vi "RSToutputWithUpDown.vi"(6 "RST Motor Constants":T1={"Pitch Gain (2*pi/enc)"=1.0, "Output Sign"=[1.0, -1.0, 1.0], "Phase Offset (rad)"=0.0, "Saturation"=32000.0}, 8 "flip Z":bool, 9 "Encoder Position":dbl, 10 "Z Command":dbl, 11 "X Command":dbl) -> (1 "Coerced?":bool, 3 "Control":dbl[](array[numeric]))   [LabVIEW 2011, in "kevLib2011.lvlib"]
uses:
  kevLib2011.lvlib
  RSTtypeDef.ctl
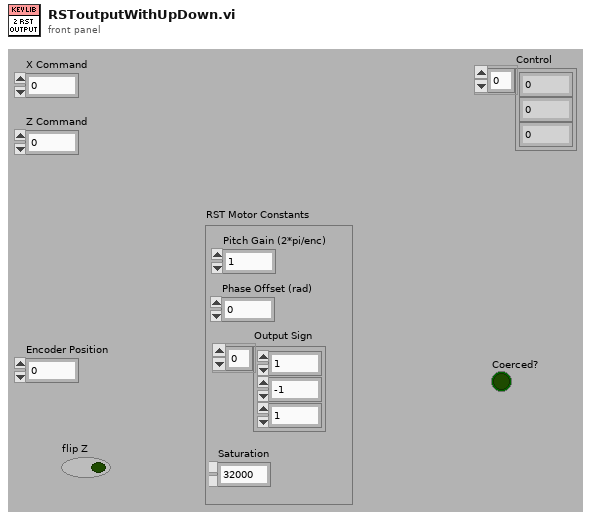
[diagram p1: front panel]
types:
  T1 = typedef "kevLib2011.lvlib/RSTtypeDef.ctl" = cluster{"Pitch Gain (2*pi/enc)":dbl, "Output Sign":dbl[], "Phase Offset (rad)":dbl, "Saturation":dbl}
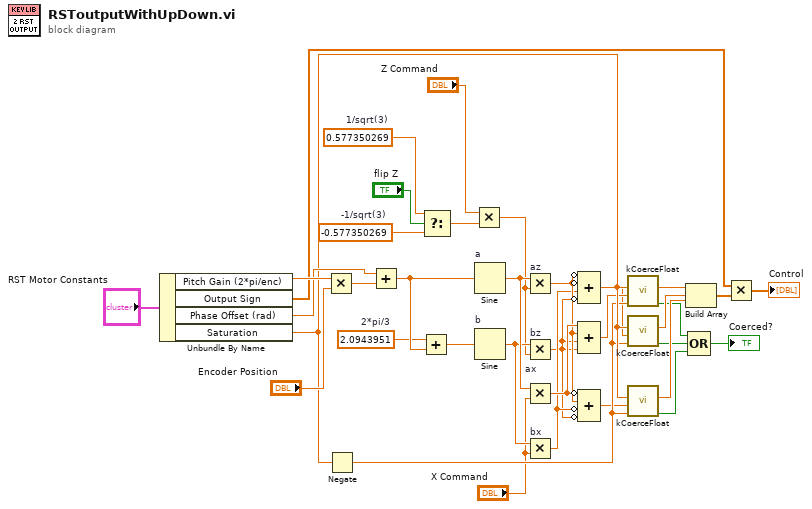
[diagram p0: block diagram]
diagram:
  w5 = -0.577350269  # -1/sqrt(3)
  w6 = 0.577350269  # 1/sqrt(3)
  w20 = 2.0943951  # 2*pi/3
  n1 = Unbundle By Name("RST Motor Constants") -> ("Pitch Gain (2*pi/enc)"=w34:dbl, "Output Sign"=w17:dbl[], "Phase Offset (rad)"=w32:dbl, "Saturation"=w24:dbl)
  n2 = Multiply(x=w34, y="Encoder Position") -> (x*y=w33:dbl)
  n3 = Negate(x=w24) -> (-x=w23:dbl)
  n4 = Add(x=w32, y=w33) -> (x+y=w22:dbl)
  n5 = Add(x=w20, y=w22) -> (x+y=w21:dbl)
  n6 = Select(t=w6, s="flip Z", f=w5) -> (s? t:f=w4:dbl)
  n7 = Multiply(x="Z Command", y=w4) -> (x*y=w12:dbl)
  n8 = Sine "a"(x=w22) -> (sin(x)=w15:dbl)
  n9 = Sine "b"(x=w21) -> (sin(x)=w14:dbl)
  n10 = Multiply "az"(x=w15, y=w12) -> (x*y=w10:dbl)
  n11 = Multiply "bz"(x=w14, y=w12) -> (x*y=w8:dbl)
  n12 = Multiply "ax"(x=w15, y="X Command") -> (x*y=w11:dbl)
  n13 = Multiply "bx"(x=w14, y="X Command") -> (x*y=w9:dbl)
  n14 = Compound Arithmetic op=ADD(invert w10, invert w10, w9, invert w8) -> (w2:dbl)
  n15 = Compound Arithmetic op=ADD(w11, w10, w8, w8) -> (w3:dbl)
  n16 = Compound Arithmetic op=ADD(invert w11, w10, invert w9, invert w8) -> (w1:dbl)
  n17 = call "kCoerceFloat.vi"("lower"=w23, "input"=w3, "upper"=w24) -> ("coerced?"=w28:bool, "output"=w31:dbl)  [unwired: 7 in]
  n18 = call "kCoerceFloat.vi"("lower"=w23, "input"=w2, "upper"=w24) -> ("coerced?"=w27:bool, "output"=w30:dbl)  [unwired: 7 in]
  n19 = call "kCoerceFloat.vi"("lower"=w23, "input"=w1, "upper"=w24) -> ("coerced?"=w26:bool, "output"=w29:dbl)  [unwired: 7 in]
  n20 = Build Array(w31, w30, w29) -> (w19:dbl[])
  n21 = Compound Arithmetic op=OR(w28, w27, w26) -> (→"Coerced?":bool)
  n22 = Multiply(x=w17, y=w19) -> (x*y=→"Control":dbl[])
